vi "FlattenByteArray.vi"(2 "Byte Array":u8[](array[numeric])) -> (4 "QWord Out":u64)   [LabVIEW 2014, in "Aquisicao de Dados.lvlib"]
uses:
  Aquisicao de Dados.lvlib
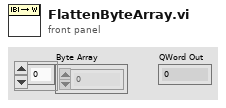
[diagram p1: front panel]
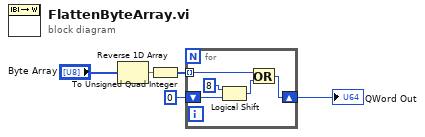
[diagram p0: block diagram]
diagram:
  n1 = Reverse 1D Array(array="Byte Array") -> (reversed array=w3:u8[])
  n2 = To Unsigned Quad Integer(1:w3) -> (0:w2:u64[])
  n3 = for {
    tunnel: w2 -> [w7] mode=indexing
    shift-right: [w9] -> w5
    shift-left: u64 0 -> [w8]
    n4 = Logical Shift(y=u32 8, x=w8) -> (x << y=w6:u64)
    n5 = Or(x=w7, y=w6) -> (x .or. y?=w9:u64)
  }
  "QWord Out" <- w5
